vi "Index Array (Object).vi"(8 "error in (no error)":errorcluster, 9 "index":i32, 11 "JSON Array in":refnum<class "JSON Array.lvclass">) -> (0 "error out":errorcluster, 2 "JSON Object":refnum<class "JSON Object.lvclass">, 3 "JSON Array out":refnum<class "JSON Array.lvclass">)   [LabVIEW 2017, in "LVJSON.lvlib" / "JSON Array.lvclass"]
uses:
  JSON Array.lvclass
  JSON Object/JSON Object.lvclass
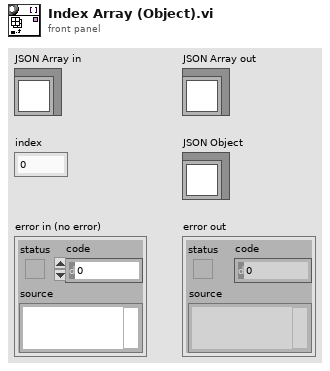
[diagram p1: front panel]
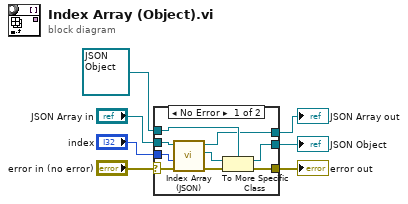
[diagram p0: block diagram]
diagram:
  n1 = case shown="No Error" "error in (no error)" {
    selector: "error in (no error)" -> [w12 w19]
    tunnel: [w8 w19] -> w6
    tunnel: [w14 w18] -> w4
    tunnel: "JSON Array in" -> [w13 w18]
    tunnel: "index" -> [w10 _]
    tunnel: [w11 w17] -> w1
    tunnel: refnum<class "JSON Object.lvclass"> refnum ("target class") -> [w15 w17]
    frame No Error {
      n2 = call "Index Array (JSON).vi"("error in (no error)"=w12, "index"=w10, "JSON Array in"=w13) -> ("error out"=w9:errorcluster, "JSON Data"=w16:refnum<class "JSON Datatype.lvclass">, "JSON Array out"=w14:refnum<class "JSON Array.lvclass">)  [unwired: 6 in]
      n3 = To More Specific Class(target class=w15, reference=w16, error in=w9) -> (specific class reference=w11:refnum<class "JSON Object.lvclass">, error out=w8:errorcluster)
    }
    frame Error {
    }
  }
  "error out" <- w6
  "JSON Array out" <- w4
  "JSON Object" <- w1
